vi "To 2D Int Tree Data.vi"(10 "2D Int":i64[][](array[numeric])) -> (3 "2D Int Tree Data":refnum<class "2D Int.lvclass">)   [LabVIEW 2017, in "Tree API.lvlib" / "2D Int.lvclass"]
doc: "Convert a 2D Int value to Tree Data type."
uses:
  2D Int.lvclass
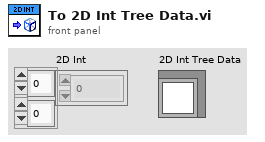
[diagram p1: front panel]
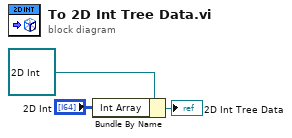
[diagram p0: block diagram]
diagram:
  n1 = Bundle By Name(cluster=refnum<class "2D Int.lvclass"> refnum ("Tree API.lvlib:2D Int.lvclass"), "Int Array"="2D Int") -> (→"2D Int Tree Data":refnum<class "2D Int.lvclass">)
